vi "WT1800 Read Measurements.vi"(0 "WT1800 Instruments In":refnum<visa-resource-name>[](array[refnum]), 1 "WT1800 Channels per Instrument":i32, 2 "WT1800 Channel Group":i32, 3 "Number of Functions":i32, 5 "Desired Functions":string[](array[string]), 11 "error in":errorcluster, 12 "Test Time has Elapsed":bool, 13 "Step Delay Time has Elapsed":bool) -> (4 "WT1800 Instruments Out":refnum<visa-resource-name>[](array[refnum]), 6 "WT1800 Measurements":sgl[][](array[numeric]), 8 "WT1800 Measurements":T2 {"Vrms" format="%.3f"; "Irms" format="%.3f"; "Power" format="%.3f"; "Vpkpk" format="%.3f"; "Ipkpk" format="%.3f"}, 10 "WT1800 Functions":T1, 15 "error out":errorcluster)   [LabVIEW 2021]
uses:
  Controls/WT1800 Measurements.ctl
  Controls/WT1800 Readings.ctl
  Controls/WT1800 Functions.ctl
panel:
  out "All Functions":string[](array[string])
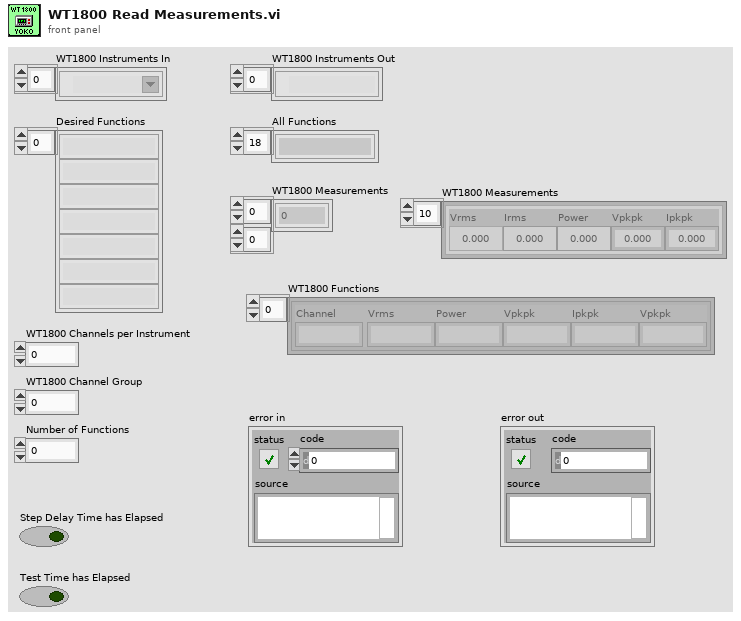
[diagram p1: front panel]
types:
  T1 = typedef "WT1800 Functions.ctl" = cluster{"Channel":string, "Vrms":string, "Power":string, "Vpkpk":string, "Ipkpk":string, "Vpkpk":string}[]
  T2 = typedef "WT1800 Measurements.ctl" = T3[]
  T3 = typedef "WT1800 Readings.ctl" = cluster{"Vrms":sgl, "Irms":sgl, "Power":sgl, "Vpkpk":sgl, "Ipkpk":sgl}
  T4 = cluster{"[0]":dbl, "[1]":dbl, "[2]":dbl, dbl, dbl}[]
  T5 = cluster{"[0]":string, "[1]":string, "[2]":string, "[3]":string, string, string}[]
  T6 = cluster{"[0]":string, "[1]":string, "[2]":string, "[3]":string, "[4]":string, "[5]":string, "[6]":string, "[7]":string}
  T7 = cluster{"[0]":dbl, "[1]":dbl, "[2]":dbl, "[3]":dbl, "[4]":dbl, "[5]":dbl, "[6]":dbl}
  T8 = cluster{"[0]":string, "[1]":string, "[2]":string, "[3]":string, "[4]":string, "[5]":string, "[6]":string, "[7]":string}[]
  T9 = cluster{"[0]":dbl, "[1]":dbl, "[2]":dbl, "[3]":dbl, "[4]":dbl, "[5]":dbl, "[6]":dbl}[]
  T10 = cluster{"[0]":dbl, "[1]":dbl, "[2]":dbl, dbl, dbl}
  T11 = cluster{"[0]":string, "[1]":string, "[2]":string, "[3]":string, string, string}
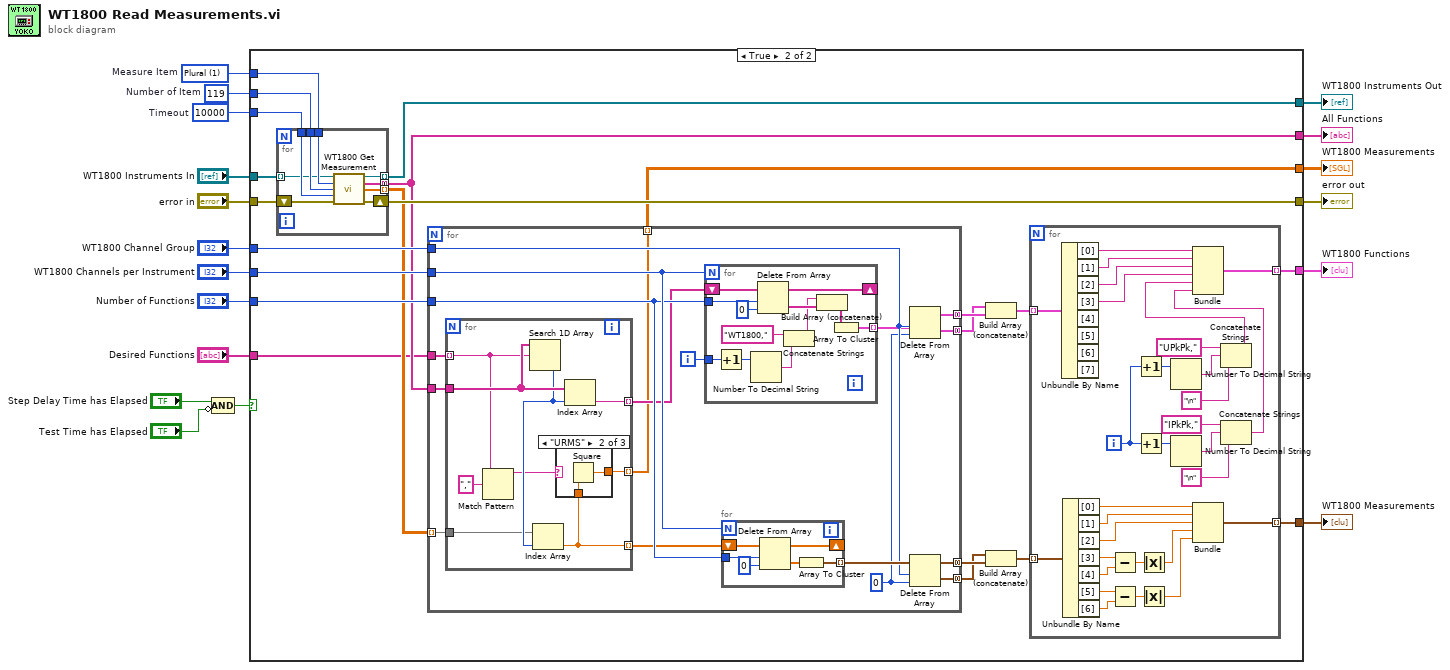
[diagram p0: block diagram]
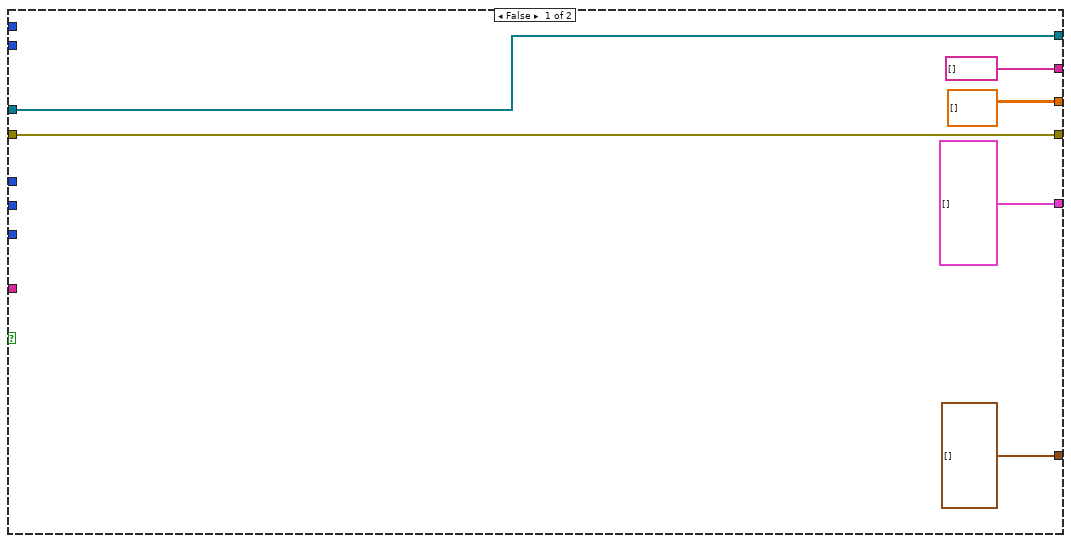
[diagram p2: hidden frame]
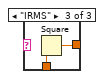
[diagram p4: hidden frame]
diagram:
  w18 = 10000  # Timeout
  w16 = 119  # Number of Item
  w17 = 1 items=["One", "Plural"]  # Measure Item
  n1 = Compound Arithmetic op=AND("Step Delay Time has Elapsed", invert "Test Time has Elapsed") -> (w3:bool)
  n2 = case shown="True" w3 {
    tunnel: w18 -> [_ w46]
    tunnel: w17 -> [_ w45]
    tunnel: w16 -> [_ w44]
    tunnel: "WT1800 Instruments In" -> [w24 w43]
    tunnel: "error in" -> [w21 w42]
    tunnel: [w21 w41] -> w1
    tunnel: [w24 w40] -> w14
    tunnel: "WT1800 Channel Group" -> [_ w35]
    tunnel: "WT1800 Channels per Instrument" -> [_ w34]
    tunnel: "Number of Functions" -> [_ w33]
    tunnel: [string[] [] ("Function") w32] -> w10
    tunnel: "Desired Functions" -> [_ w25]
    tunnel: [T5 [] w28] -> w8
    tunnel: [T4 [] w27] -> w7
    tunnel: [dbl[][] [] w26] -> w6
    frame False {
    }
    frame True {
      n3 = for {
        tunnel: w46 -> [w134]
        tunnel: w45 -> [w133]
        tunnel: w44 -> [w132]
        tunnel: [w130] -> w40 mode=indexing
        tunnel: [w126] -> w32 mode=concatenating
        tunnel: [w129] -> w31 mode=indexing
        tunnel: w43 -> [w128] mode=indexing
        shift-right: [w131] -> w41
        shift-left: w42 -> [w127]
        n4 = call "WT1800 Get Measurement.vi"("VISA resource name"=w128, "Measure Item (1: Plural)"=w133, "Number of Item (15)"=w132, "Timeout (10000 ms)"=w134, "error in (no error)"=w127) -> ("VISA resource name out"=w130:refnum<visa-resource-name>, "Function"=w126:string[], "Measurement"=w129:dbl[], "error out"=w131:errorcluster)  [unwired: 7 in]
      }
      n5 = for {
        tunnel: w25 -> [w93]
        tunnel: w32 -> [w92]
        tunnel: w33 -> [w82]
        tunnel: w34 -> [w83]
        tunnel: [w90] -> w39 mode=concatenating
        tunnel: [w91] -> w38 mode=concatenating
        tunnel: w35 -> [w87]
        tunnel: w31 -> [w89] mode=indexing
        tunnel: [w85] -> w37 mode=concatenating
        tunnel: [w84] -> w36 mode=concatenating
        tunnel: [w77] -> w26 mode=indexing
        i -> [w79]
        w86 = 0 ("index")
        n6 = for {
          tunnel: w92 -> [w119]
          tunnel: w93 -> [w113] mode=indexing
          tunnel: [w120] -> w81 mode=indexing
          tunnel: w89 -> [w117]
          tunnel: [w115] -> w78 mode=indexing
          tunnel: [w116] -> w77 mode=indexing
          n7 = Match Pattern(string=w113, regular expression=",") -> (before substring=w112:string)  [unwired: 1 in, 3 out]
          n8 = Search 1D Array(1D array=w119, element=w113) -> (index of element=w118:i32)  [unwired: 1 in]
          n9 = Index Array(array=w117, index=w118) -> (element=w115:dbl)
          n10 = case shown="\"URMS\"" w112 {
            tunnel: w115 -> [w121 w123 w125]
            tunnel: [w121 w122 w124] -> w116
            frame "", Default {
            }
            frame "URMS" {
              n11 = Square(x=w123) -> (x^2=w122:dbl)
            }
            frame "IRMS" {
              n12 = Square(x=w125) -> (x^2=w124:dbl)
            }
          }
          n13 = Index Array(array=w119, index=w118) -> (element=w120:string)
        }
        n14 = for {
          N: w83 -> [_]
          shift-right: [w104] -> _
          shift-left: w81 -> [w105]
          tunnel: w82 -> [w103]
          tunnel: [w101] -> w80 mode=indexing
          tunnel: w79 -> [w96]
          n15 = Increment(x=w96) -> (x+1=w99:i32)
          n16 = Number To Decimal String(number=w99) -> (decimal integer string=w98:string)  [unwired: 1 in]
          n17 = Delete From Array(array=w105, length=w103, index=0) -> (deleted portion=w95:string[], array with subset deleted=w104:string[])
          n18 = Concatenate Strings("WT1800," ("string"), w98) -> (w94:string)
          n19 = Build Array (concatenate)(w94, w95) -> (w97:string[])
          n20 = Array To Cluster(array=w97) -> (cluster=w101:T6)
        }
        n21 = for {
          N: w83 -> [_]
          shift-right: [w110] -> _
          shift-left: w78 -> [w111]
          tunnel: w82 -> [w109]
          tunnel: [w106] -> w88 mode=indexing
          n22 = Delete From Array(array=w111, length=w109, index=0) -> (deleted portion=w108:dbl[], array with subset deleted=w110:dbl[])
          n23 = Array To Cluster(array=w108) -> (cluster=w106:T7)
        }
        n24 = Delete From Array(array=w80, length=w87, index=w86) -> (deleted portion=w91:T8, array with subset deleted=w90:T8)
        n25 = Delete From Array(array=w88, length=w87, index=w86) -> (deleted portion=w84:T9, array with subset deleted=w85:T9)
      }
      n26 = Build Array (concatenate)(w38, w39) -> (w30:T8)
      n27 = Build Array (concatenate)(w36, w37) -> (w29:T9)
      n28 = for {
        tunnel: w30 -> [w76] mode=indexing
        tunnel: w29 -> [w75] mode=indexing
        tunnel: [w59] -> w28 mode=indexing
        tunnel: [w58] -> w27 mode=indexing
        i -> [w47]
        n29 = Unbundle By Name(w76) -> ("[0]"=w64:string, "[1]"=w63:string, "[2]"=w62:string, "[3]"=w61:string)  [unwired: 4 out]
        n30 = Unbundle By Name(w75) -> ("[0]"=w69:dbl, "[1]"=w68:dbl, "[2]"=w67:dbl, "[3]"=w71:dbl, "[4]"=w70:dbl, "[5]"=w74:dbl, "[6]"=w60:dbl)
        n31 = Subtract(x=w71, y=w70) -> (x-y=w72:dbl)
        n32 = Subtract(x=w74, y=w60) -> (x-y=w73:dbl)
        n33 = Increment(x=w47) -> (x+1=w56:i32)
        n34 = Increment(x=w47) -> (x+1=w51:i32)
        n35 = Absolute Value(x=w72) -> (abs(x)=w66:dbl)
        n36 = Absolute Value(x=w73) -> (abs(x)=w65:dbl)
        n37 = Number To Decimal String(number=w56) -> (decimal integer string=w57:string)  [unwired: 1 in]
        n38 = Number To Decimal String(number=w51) -> (decimal integer string=w50:string)  [unwired: 1 in]
        n39 = Bundle("[0]"=w69, "[1]"=w68, "[2]"=w67, w66, w65) -> (w58:T10)  [unwired: 1 in]
        n40 = Concatenate Strings("UPkPk," ("string"), w57, "\n" ("[4]")) -> (w48:string)
        n41 = Concatenate Strings("IPkPk," ("string"), w50, "\n" ("[4]")) -> (w49:string)
        n42 = Bundle("[0]"=w64, "[1]"=w63, "[2]"=w62, "[3]"=w61, w48, w49) -> (w59:T11)  [unwired: 1 in]
      }
    }
  }
  "WT1800 Instruments Out" <- w14
  "WT1800 Measurements" <- w6
  "All Functions" <- w10
  "WT1800 Measurements" <- w7
  "WT1800 Functions" <- w8
  "error out" <- w1
